vi "Token Type Equals.vi"(2 "Type":T1, 3 "Token":T2) -> (0 "Type Equals?":bool)   [LabVIEW 2020, in "Stream.lvlib" / "URLPattern.lvclass"]
uses:
  URLPattern.lvclass
  Token.ctl
  Token Type.ctl
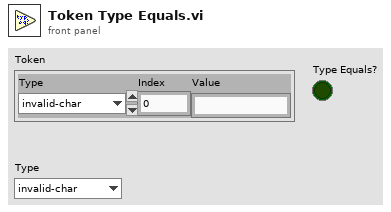
[diagram p1: front panel]
types:
  T1 = typedef "Stream.lvlib/URLPattern.lvclass/Token Type.ctl" = enum16{"invalid-char", "open", "close", "regexp", "name", "char", "escaped-char", "other-modifier", "asterisk", "end"}
  T2 = typedef "Stream.lvlib/URLPattern.lvclass/Token.ctl" = cluster{"Type":T1, "Index":i32, "Value":string}
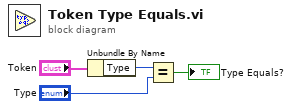
[diagram p0: block diagram]
diagram:
  n1 = Unbundle By Name("Token") -> ("Type"=w4:T1)
  n2 = Equal?(x=w4, y="Type") -> (x = y?=→"Type Equals?":bool)
